vi "Configure Histogram.vi"(6 "Enable Histogram Auto Range (False)":bool, 7 "Histogram Range (0.0)":dbl format="%^.3e", 8 "error in (no error)":errorcluster {"code" format="%.0x"}, 9 "Enable Histogram (False)":bool, 10 "Channel Name (1)":string="1", 11 "VISA resource name":refnum<visa-resource-name>) -> (0 "error out":errorcluster {"code" format="%.0x"}, 3 "VISA resource name out":refnum<visa-resource-name>)   [LabVIEW 2010, in "Agilent N6700 Series.lvlib"]
doc: "This VI configures the histogram function.\n\n<b>Note:</b>\n\n(1) This VI only applies to models N6781A and N6782A that have the Data Logger function installed.\n\n(2) The histogram function only applies to the N6705B DC Power Analyzer."
uses:
  Agilent N6700 Series.lvlib
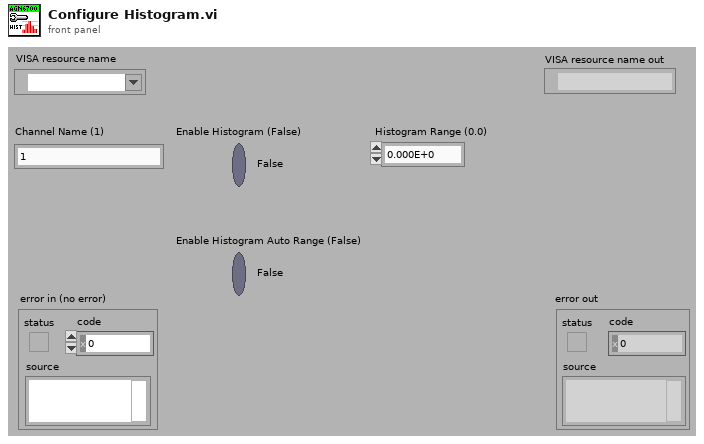
[diagram p1: front panel]
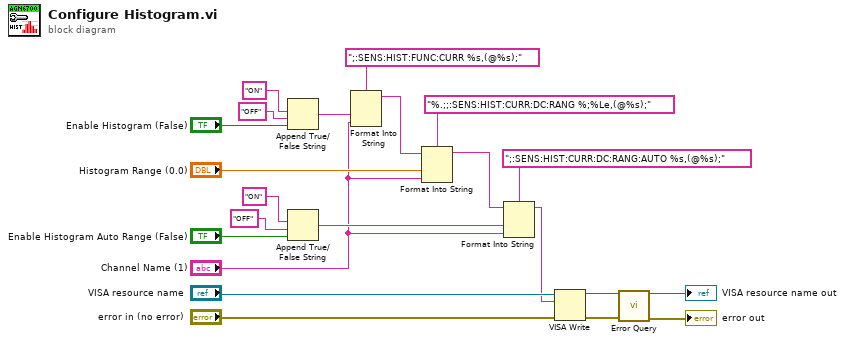
[diagram p0: block diagram]
diagram:
  n1 = Append True/False String(1:"Enable Histogram (False)", 2:"OFF", 3:"ON") -> (0:w8:string)  [unwired: 1 in]
  n2 = Append True/False String(1:"Enable Histogram Auto Range (False)", 2:"OFF", 3:"ON") -> (0:w5:string)  [unwired: 1 in]
  n3 = Format Into String(format string=";:SENS:HIST:FUNC:CURR %s,(@%s);", w8, "Channel Name (1)") -> (resulting string=w13:string)  [unwired: 2 in, 1 out]
  n4 = Format Into String(format string="%.;;:SENS:HIST:CURR:DC:RANG %;%Le,(@%s);", initial string=w13, "Histogram Range (0.0)", "Channel Name (1)") -> (resulting string=w16:string)  [unwired: 1 in, 1 out]
  n5 = Format Into String(format string=";:SENS:HIST:CURR:DC:RANG:AUTO %s,(@%s);", initial string=w16, w5, "Channel Name (1)") -> (resulting string=w14:string)  [unwired: 1 in, 1 out]
  n6 = VISA Write(VISA resource name="VISA resource name", write buffer=w14, error in (no error)="error in (no error)") -> (VISA resource name out=w18:refnum<visa-resource-name>, error out=w17:errorcluster)  [unwired: 1 out]
  n7 = call "Error Query.vi"("VISA resource name"=w18, "error in (no error)"=w17) -> ("VISA resource name out"=→"VISA resource name out":refnum<visa-resource-name>, "error out"=→"error out":errorcluster)  [unwired: 10 in, 2 out]
